vi "AutoSetPreSetPos.vi"(8 "error in (no error)":errorcluster, 10 "Game Piece":enum16{"Cube", "Cone"}(ring), 11 "Position":enum16{"Upper", "Lower", "Middle"}(ring)) -> (0 "error out":errorcluster)   [LabVIEW 2020]
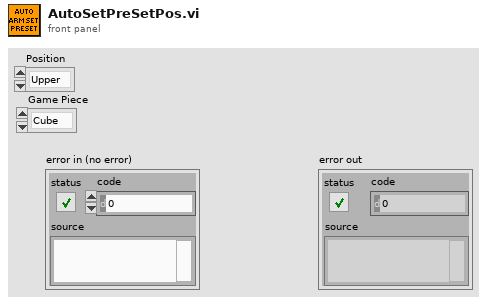
[diagram p1: front panel]
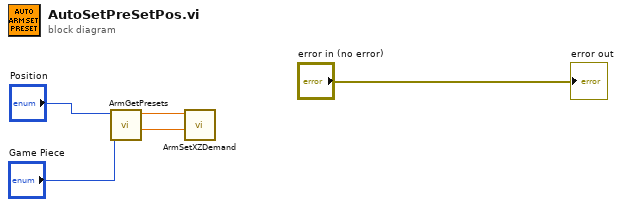
[diagram p0: block diagram]
diagram:
  n1 = call "ArmGetPresets.vi"("Game Piece"="Game Piece", "Position"="Position") -> ("z"=w3:dbl, "x"=w4:dbl)  [unwired: 8 in]
  n2 = call "ArmSetXZDemand.vi"("SetZ"=w3, "SetX"=w4) -> ()  [unwired: 10 in]
  "error out" <- "error in (no error)"
